vi "GetRGB.vi"(0 "ColorRGB in":refnum<class "ColorRGB.lvclass">, 11 "error in (no error)":errorcluster) -> (4 "ColorRGB out":refnum<class "ColorRGB.lvclass">, 6 "R":u8, 8 "G":u8, 10 "B":u8, 15 "error out":errorcluster)   [LabVIEW 2021, in "Picture2D.lvlib" / "ColorRGB.lvclass"]
uses:
  ColorRGB.lvclass
  C:/GitHub/Picture2D/src/Color/Color.lvclass
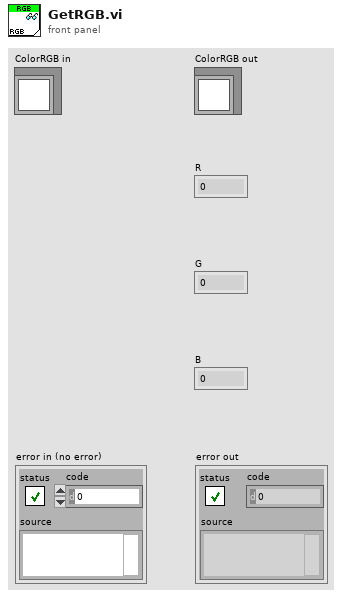
[diagram p1: front panel]
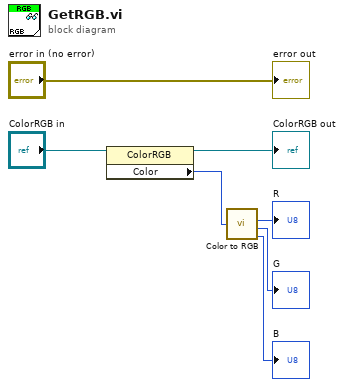
[diagram p0: block diagram]
diagram:
  n1 = property class="ColorRGB"(reference="ColorRGB in") -> (reference out=→"ColorRGB out":refnum<class "ColorRGB.lvclass">, "Color"=w1:u32)  [unwired: 1 in, 1 out]
  n2 = call <vilib>:"Color to RGB.vi"("Color"=w1) -> ("R"=→"R":u8, "G"=→"G":u8, "B"=→"B":u8)  [unwired: 1 out]
  "error out" <- "error in (no error)"
